vi "InsertSN.vi"(10 "SN":u32 format="%.0x", 11 "Full Text File In":u8[](array[numeric]) format="%.0x") -> (2 "Full Text File Out":u8[](array[numeric]) format="%.0x")   [LabVIEW 2017]
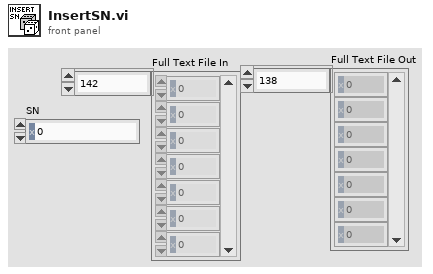
[diagram p1: front panel]
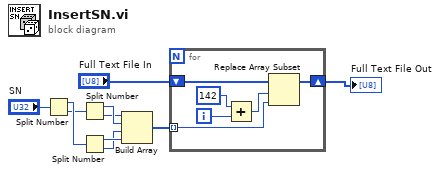
[diagram p0: block diagram]
diagram:
  n1 = Split Number(x="SN") -> (hi(x)=w9:u16, lo(x)=w8:u16)
  n2 = Split Number(x=w8) -> (hi(x)=w5:u8, lo(x)=w4:u8)
  n3 = Split Number(x=w9) -> (hi(x)=w7:u8, lo(x)=w6:u8)
  n4 = Build Array(w4, w5, w6, w7) -> (w3:u8[])
  n5 = for {
    shift-right: [w15] -> w1
    shift-left: "Full Text File In" -> [w16]
    tunnel: w3 -> [w14] mode=indexing
    i -> [w11]
    n6 = Add(x=142 ("index"), y=w11) -> (x+y=w12:i32)
    n7 = Replace Array Subset(array=w16, new element=w14, index=w12) -> (w15:u8[])
  }
  "Full Text File Out" <- w1
